vi "菜单-打开.vi"(8 "error in (no error)":errorcluster caption="错误输入（无错误）", 11 "程序响应 输入":refnum<class "程序响应.lvclass">) -> (0 "error out":errorcluster caption="错误输出", 3 "程序响应 输出":refnum<class "程序响应.lvclass">)   [LabVIEW 2020, in "程序响应.lvlib" / "程序响应.lvclass"]
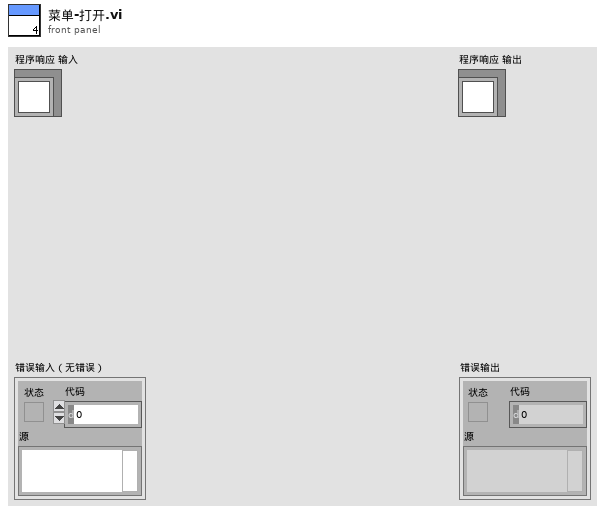
[diagram p1: front panel]
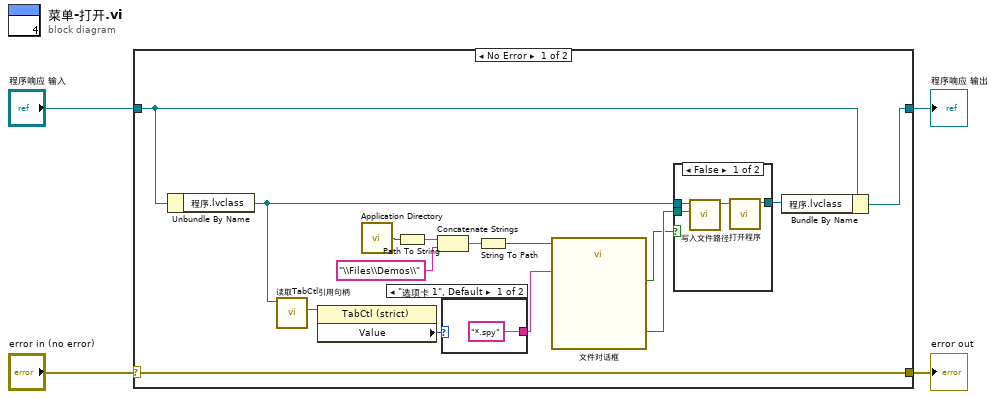
[diagram p0: block diagram]
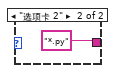
[diagram p3: hidden frame]
diagram:
  n1 = case shown="No Error" "error in (no error)" {
    selector: "error in (no error)" -> [w19 w28]
    tunnel: [w19 w28] -> w3
    tunnel: [w16 w27] -> w1
    tunnel: "程序响应 输入" -> [w17 w27]
    frame No Error {
      n2 = Unbundle By Name(w17) -> ("程序.lvclass"=w9:refnum<class "程序.lvclass">)
      n3 = call-dynamic "读取TabCtl引用句柄.vi"("程序输入"=w9) -> ("TabCtl引用句柄"=w8:refnum<vi>)  [unwired: 8 in, 2 out]
      n4 = property class="TabCtl (strict)"(reference=w8) -> ("Value"=w7:enum32{"选项卡 1", "选项卡 2"})  [unwired: 1 in, 2 out]
      n5 = call <vilib>:"Application Directory.vi"() -> ("Application Directory"=w11:path)
      n6 = Path To String(path=w11) -> (string=w14:string)
      n7 = Concatenate Strings(w14, "\\Files\\Demos\\" ("名称或相对路径")) -> (w13:string)
      n8 = case shown="\"选项卡 1\", Default" w7 {
        tunnel: ["*.spy" ("pattern (all files)") "*.py" ("pattern (all files)")] -> w6
        frame "选项卡 1", Default {
        }
        frame "选项卡 2" {
        }
      }
      n9 = String To Path(string=w13) -> (path=w10:path)
      n10 = call "文件对话框"("start path"=w10, "pattern (all files)"=w6) -> ("selected path"=w15:path, "cancelled"=w5:bool)  [unwired: 10 in, 2 out]
      n11 = case shown="False" w5 {
        tunnel: [w23 w24] -> w18
        tunnel: w15 -> [w21 _]
        tunnel: w9 -> [w20 w24]
        frame False {
          n12 = call-dynamic "写入文件路径.vi"("文件路径"=w21, "程序输入"=w20) -> ("程序输出"=w22:refnum<class "程序.lvclass">)  [unwired: 8 in, 1 out]
          n13 = call-dynamic "打开程序.vi"("程序 输入"=w22) -> ("程序 输出"=w23:refnum<class "程序.lvclass">)  [unwired: 9 in, 1 out]
        }
        frame True {
        }
      }
      n14 = Bundle By Name(cluster=w17, "程序.lvclass"=w18) -> (w16:refnum<class "程序响应.lvclass">)
    }
    frame Error {
    }
  }
  "error out" <- w3
  "程序响应 输出" <- w1
